vi "Pockels Cal-Objective cal start actions.vi"(11 "Objective index":i32) -> (0 "error out":errorcluster, 3 "Cancelled (Left button pressed)":bool)   [LabVIEW 2013]
uses:
  Globals/gl_Calibration globals.vi
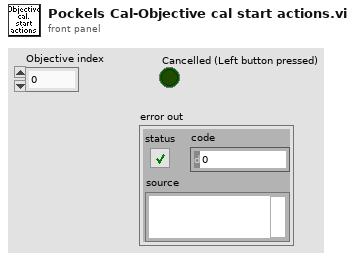
[diagram p1: front panel]
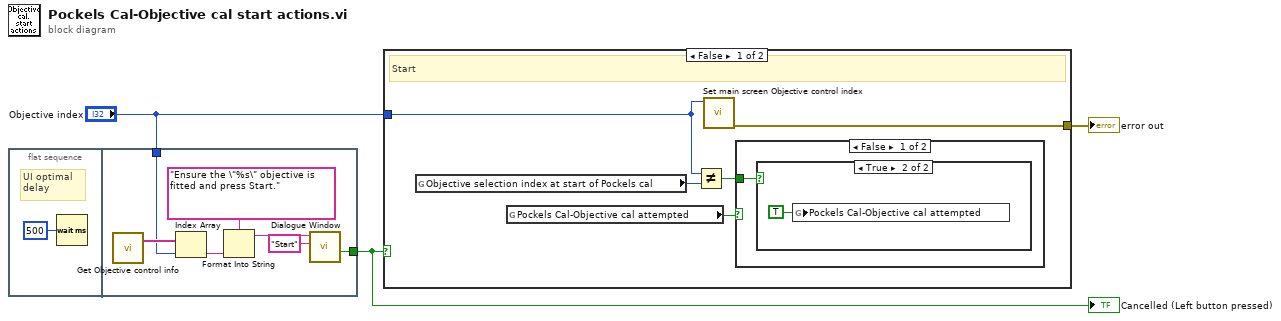
[diagram p0: block diagram]
diagram:
  n1 = flat-sequence {
    tunnel: [w11] -> w1
    tunnel: "Objective index" -> [w5]
    frame #0 {
      # "UI optimal delay"
      n2 = Wait (ms)(milliseconds to wait=u32 500) -> ()  [unwired: 1 out]
    }
    frame #1 {
      n3 = call "Get Objective control info.vi"() -> ("Objective values/strings"=w10:string[])  [unwired: 7 in, 4 out]
      n4 = Index Array(array=w10, index=w5) -> (element=w7:string)
      n5 = Format Into String(format string="Ensure the \"%s\" objective is fitted and press Start.", w7) -> (resulting string=w8:string)  [unwired: 2 in, 1 out]
      n6 = call "Dialogue Window.vi"("Caption-Right button (OK)"="Start", "Message string"=w8) -> ("Cancelled (Left button pressed)"=w11:bool)  [unwired: 7 in, 2 out]
    }
  }
  n7 = case shown="False" w1 {
    tunnel: [w16 _] -> w3
    tunnel: "Objective index" -> [w12 _]
    frame False {
      # "Start"
      n8 = global read "gl_Calibration globals.vi" "Objective selection index at start of Pockels cal"() -> (w15:i32)
      n9 = global read "gl_Calibration globals.vi" "Pockels Cal-Objective cal attempted"() -> (w14:bool)
      n10 = Not Equal?(x=w12, y=w15) -> (x != y?=w13:bool)
      n11 = call "Set main screen Objective control index.vi"("Objective control index"=w12) -> ("error out"=w16:errorcluster)  [unwired: 9 in, 1 out]
      n12 = case shown="False" w14 {
        tunnel: w13 -> [w17 _]
        frame False {
          n13 = case shown="True" w17 {
            frame False {
            }
            frame True {
              n14 = global write "gl_Calibration globals.vi" "Pockels Cal-Objective cal attempted"(TRUE ("Pockels Cal-Objective cal attempted")) -> ()
            }
          }
        }
        frame True {
        }
      }
    }
    frame True {
      # "Cancelled"
    }
  }
  "error out" <- w3
  "Cancelled (Left button pressed)" <- w1
